vi "Pixie4ReadRunStatistics.vi"(8 "error in (no error)":errorcluster) -> (0 "error out":errorcluster, 2 "Run time [s]":dbl, 3 "run data output":T1, 5 "number of events":dbl)   [LabVIEW 2016]
uses:
  Drivers/Pixie4DLL.dll
panel:
  in  "run data":T1
  in  "Module number":u16 max=17 step=1
  in  "Run statistics":enum32{"Channel", "Module"}(tab)
  out "GDT3":dbl
  out "GDT2":dbl
  out "GDT1":dbl
  out "GDT0":dbl
  out "GateRate3":dbl
  out "GateRate2":dbl
  out "GateRate1":dbl
  out "GateRate0":dbl
  out "SFDT3":dbl
  out "SFDT2":dbl
  out "SFDT1":dbl
  out "SFDT0":dbl
  out "OCR3":dbl
  out "OCR2":dbl
  out "OCR1":dbl
  out "OCR0":dbl
  out "ICR3":dbl
  out "ICR2":dbl
  out "ICR1":dbl
  out "ICR0":dbl
  out "LT3":dbl
  out "LT2":dbl
  out "LT1":dbl
  out "LT0":dbl
  out "Total time [s]":dbl
  out "Event rate [cps]":dbl
  out "x/y":dbl
  # "Channel"
  # "Live time [s]"
  # "Input rates [cps]"
  # "Output rates [cps]"
  # "Filter dead time [s]"
  # "Gate rate [cps]"
  # "Gate dead time [s]"
  # "0"
  # "1"
  # "2"
  # "3"
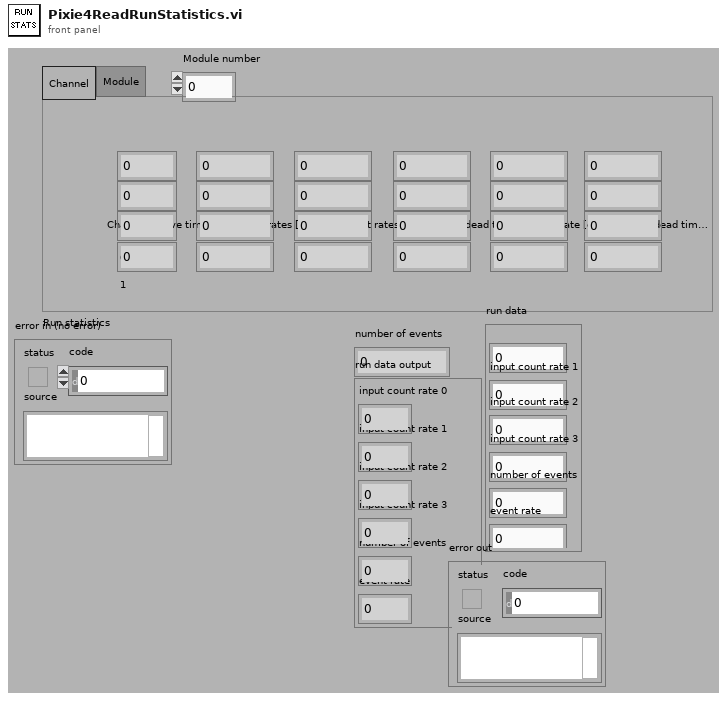
[diagram p1: front panel]
types:
  T1 = cluster{"input count rate 0":dbl, "input count rate 1":dbl, "input count rate 2":dbl, "input count rate 3":dbl, "number of events":dbl, "event rate":dbl}
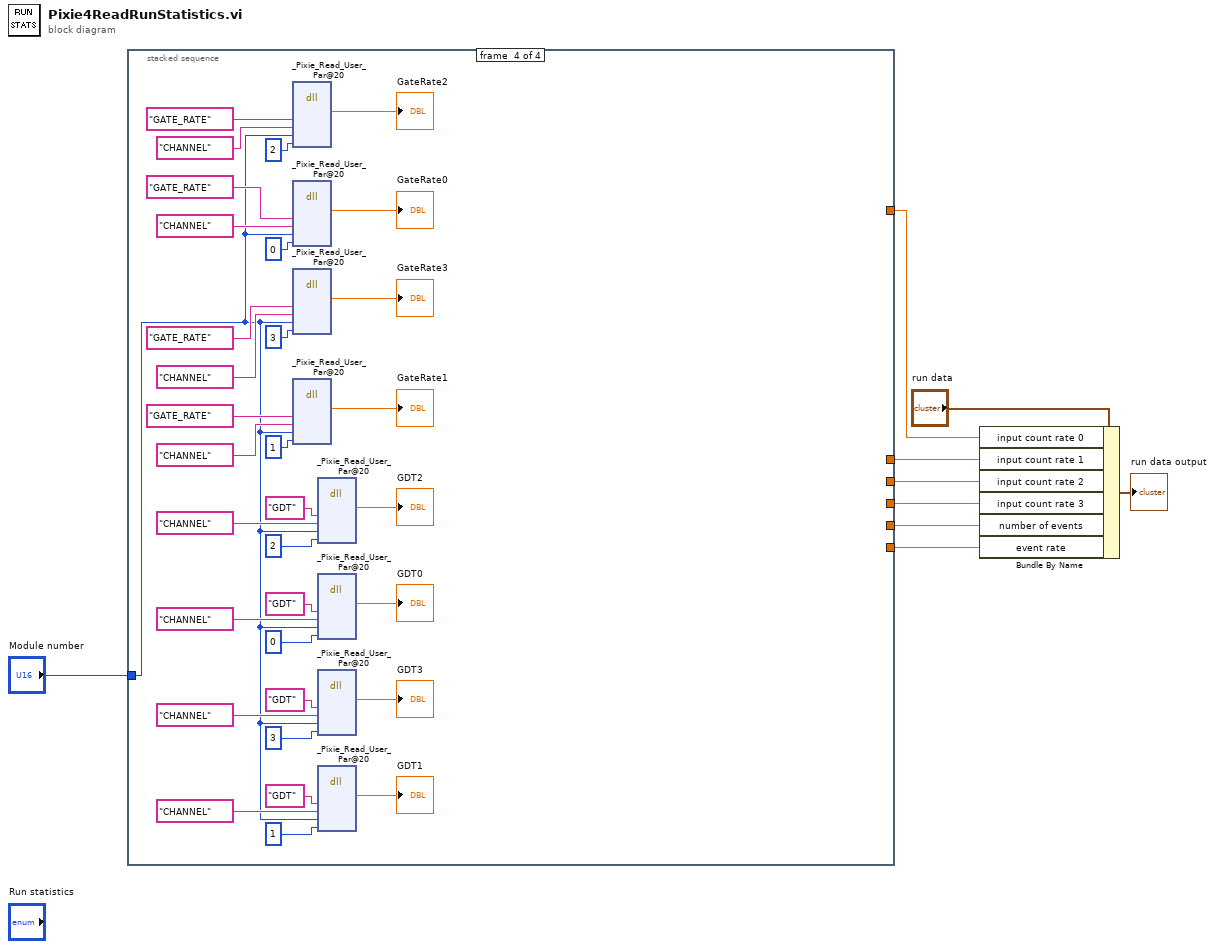
[diagram p0: block diagram]
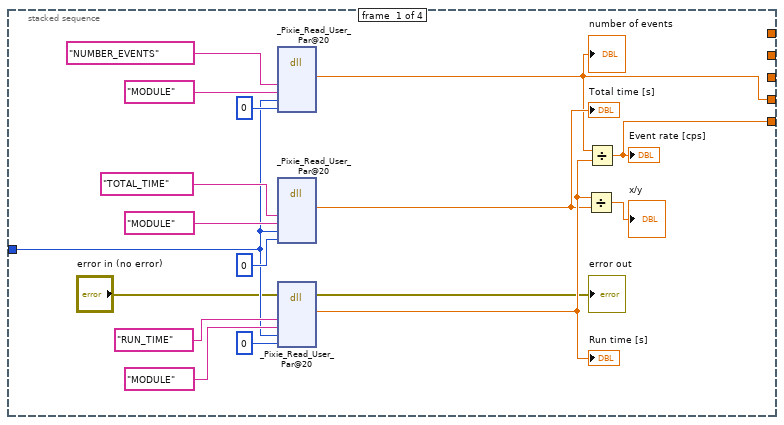
[diagram p2: hidden frame]
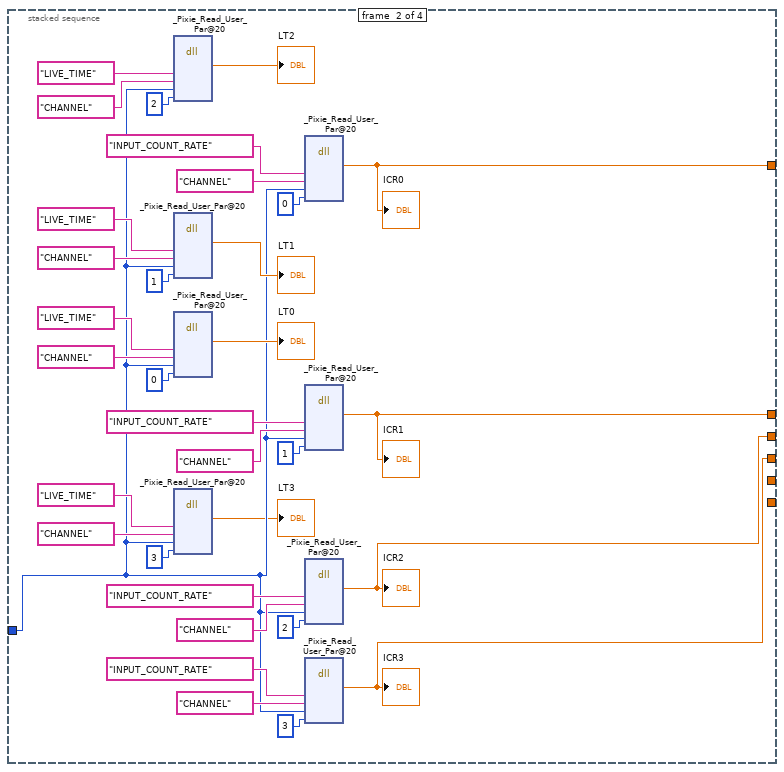
[diagram p3: hidden frame]
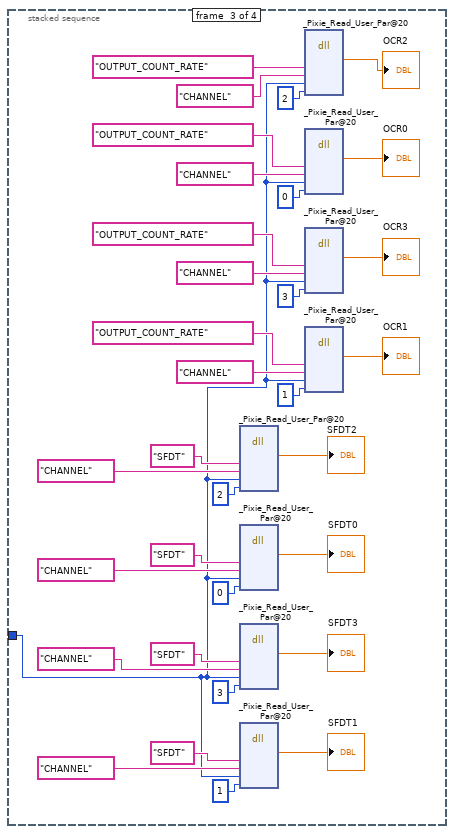
[diagram p4: hidden frame]
diagram:
  n1 = stacked-sequence {
    tunnel: "Module number" -> [w17 w32 w60 w93]
    tunnel: [_ w30 _ _] -> w7
    tunnel: [_ w29 _ _] -> w6
    tunnel: [_ w28 _ _] -> w5
    tunnel: [_ w27 _ _] -> w4
    tunnel: [w13 _ _ _] -> w3
    tunnel: [w12 _ _ _] -> w2
    frame #0 {
      n2 = dll-call lib="D:/Users/wymanm/Desktop/DAQuiri - 2017a/lois/Drivers/Pixie4DLL.dll" fn="_Pixie_Read_User_Par@20"("User_Par_Name"="NUMBER_EVENTS", "User_Par_Type"="MODULE", "ModNum"=w17, "ChanNum"=0) -> ("User_Par_Value"=w13:dbl)  [unwired: 9 in, 2 out]
      "number of events" <- w13
      n3 = dll-call lib="D:/Users/wymanm/Desktop/DAQuiri - 2017a/lois/Drivers/Pixie4DLL.dll" fn="_Pixie_Read_User_Par@20"("User_Par_Name"="TOTAL_TIME", "User_Par_Type"="MODULE", "ModNum"=w17, "ChanNum"=0) -> ("User_Par_Value"=w15:dbl)  [unwired: 9 in, 2 out]
      "Total time [s]" <- w15
      n4 = dll-call lib="D:/Users/wymanm/Desktop/DAQuiri - 2017a/lois/Drivers/Pixie4DLL.dll" fn="_Pixie_Read_User_Par@20"(error in="error in (no error)", "User_Par_Name"="RUN_TIME", "User_Par_Type"="MODULE", "ModNum"=w17, "ChanNum"=0) -> (error out=→"error out":errorcluster, "User_Par_Value"=w16:dbl)  [unwired: 8 in, 1 out]
      "Run time [s]" <- w16
      n5 = Divide(x=w16, y=w15) -> (x/y=→"x/y":dbl)
      n6 = Divide(x=w13, y=w16) -> (x/y=w12:dbl)
      "Event rate [cps]" <- w12
    }
    frame #1 {
      n7 = dll-call lib="D:/Users/wymanm/Desktop/DAQuiri - 2017a/lois/Drivers/Pixie4DLL.dll" fn="_Pixie_Read_User_Par@20"("User_Par_Name"="LIVE_TIME", "User_Par_Type"="CHANNEL", "ModNum"=w32, "ChanNum"=2) -> ("User_Par_Value"=→"LT2":dbl)  [unwired: 9 in, 2 out]
      n8 = dll-call lib="D:/Users/wymanm/Desktop/DAQuiri - 2017a/lois/Drivers/Pixie4DLL.dll" fn="_Pixie_Read_User_Par@20"("User_Par_Name"="LIVE_TIME", "User_Par_Type"="CHANNEL", "ModNum"=w32, "ChanNum"=1) -> ("User_Par_Value"=→"LT1":dbl)  [unwired: 9 in, 2 out]
      n9 = dll-call lib="D:/Users/wymanm/Desktop/DAQuiri - 2017a/lois/Drivers/Pixie4DLL.dll" fn="_Pixie_Read_User_Par@20"("User_Par_Name"="LIVE_TIME", "User_Par_Type"="CHANNEL", "ModNum"=w32, "ChanNum"=0) -> ("User_Par_Value"=→"LT0":dbl)  [unwired: 9 in, 2 out]
      n10 = dll-call lib="D:/Users/wymanm/Desktop/DAQuiri - 2017a/lois/Drivers/Pixie4DLL.dll" fn="_Pixie_Read_User_Par@20"("User_Par_Name"="LIVE_TIME", "User_Par_Type"="CHANNEL", "ModNum"=w32, "ChanNum"=3) -> ("User_Par_Value"=→"LT3":dbl)  [unwired: 9 in, 2 out]
      n11 = dll-call lib="D:/Users/wymanm/Desktop/DAQuiri - 2017a/lois/Drivers/Pixie4DLL.dll" fn="_Pixie_Read_User_Par@20"("User_Par_Name"="INPUT_COUNT_RATE", "User_Par_Type"="CHANNEL", "ModNum"=w32, "ChanNum"=0) -> ("User_Par_Value"=w30:dbl)  [unwired: 9 in, 2 out]
      "ICR0" <- w30
      n12 = dll-call lib="D:/Users/wymanm/Desktop/DAQuiri - 2017a/lois/Drivers/Pixie4DLL.dll" fn="_Pixie_Read_User_Par@20"("User_Par_Name"="INPUT_COUNT_RATE", "User_Par_Type"="CHANNEL", "ModNum"=w32, "ChanNum"=1) -> ("User_Par_Value"=w29:dbl)  [unwired: 9 in, 2 out]
      "ICR1" <- w29
      n13 = dll-call lib="D:/Users/wymanm/Desktop/DAQuiri - 2017a/lois/Drivers/Pixie4DLL.dll" fn="_Pixie_Read_User_Par@20"("User_Par_Name"="INPUT_COUNT_RATE", "User_Par_Type"="CHANNEL", "ModNum"=w32, "ChanNum"=2) -> ("User_Par_Value"=w28:dbl)  [unwired: 9 in, 2 out]
      "ICR2" <- w28
      n14 = dll-call lib="D:/Users/wymanm/Desktop/DAQuiri - 2017a/lois/Drivers/Pixie4DLL.dll" fn="_Pixie_Read_User_Par@20"("User_Par_Name"="INPUT_COUNT_RATE", "User_Par_Type"="CHANNEL", "ModNum"=w32, "ChanNum"=3) -> ("User_Par_Value"=w27:dbl)  [unwired: 9 in, 2 out]
      "ICR3" <- w27
    }
    frame #2 {
      n15 = dll-call lib="D:/Users/wymanm/Desktop/DAQuiri - 2017a/lois/Drivers/Pixie4DLL.dll" fn="_Pixie_Read_User_Par@20"("User_Par_Name"="SFDT", "User_Par_Type"="CHANNEL", "ModNum"=w60, "ChanNum"=2) -> ("User_Par_Value"=→"SFDT2":dbl)  [unwired: 9 in, 2 out]
      n16 = dll-call lib="D:/Users/wymanm/Desktop/DAQuiri - 2017a/lois/Drivers/Pixie4DLL.dll" fn="_Pixie_Read_User_Par@20"("User_Par_Name"="SFDT", "User_Par_Type"="CHANNEL", "ModNum"=w60, "ChanNum"=0) -> ("User_Par_Value"=→"SFDT0":dbl)  [unwired: 9 in, 2 out]
      n17 = dll-call lib="D:/Users/wymanm/Desktop/DAQuiri - 2017a/lois/Drivers/Pixie4DLL.dll" fn="_Pixie_Read_User_Par@20"("User_Par_Name"="SFDT", "User_Par_Type"="CHANNEL", "ModNum"=w60, "ChanNum"=3) -> ("User_Par_Value"=→"SFDT3":dbl)  [unwired: 9 in, 2 out]
      n18 = dll-call lib="D:/Users/wymanm/Desktop/DAQuiri - 2017a/lois/Drivers/Pixie4DLL.dll" fn="_Pixie_Read_User_Par@20"("User_Par_Name"="SFDT", "User_Par_Type"="CHANNEL", "ModNum"=w60, "ChanNum"=1) -> ("User_Par_Value"=→"SFDT1":dbl)  [unwired: 9 in, 2 out]
      n19 = dll-call lib="D:/Users/wymanm/Desktop/DAQuiri - 2017a/lois/Drivers/Pixie4DLL.dll" fn="_Pixie_Read_User_Par@20"("User_Par_Name"="OUTPUT_COUNT_RATE", "User_Par_Type"="CHANNEL", "ModNum"=w60, "ChanNum"=2) -> ("User_Par_Value"=→"OCR2":dbl)  [unwired: 9 in, 2 out]
      n20 = dll-call lib="D:/Users/wymanm/Desktop/DAQuiri - 2017a/lois/Drivers/Pixie4DLL.dll" fn="_Pixie_Read_User_Par@20"("User_Par_Name"="OUTPUT_COUNT_RATE", "User_Par_Type"="CHANNEL", "ModNum"=w60, "ChanNum"=0) -> ("User_Par_Value"=→"OCR0":dbl)  [unwired: 9 in, 2 out]
      n21 = dll-call lib="D:/Users/wymanm/Desktop/DAQuiri - 2017a/lois/Drivers/Pixie4DLL.dll" fn="_Pixie_Read_User_Par@20"("User_Par_Name"="OUTPUT_COUNT_RATE", "User_Par_Type"="CHANNEL", "ModNum"=w60, "ChanNum"=3) -> ("User_Par_Value"=→"OCR3":dbl)  [unwired: 9 in, 2 out]
      n22 = dll-call lib="D:/Users/wymanm/Desktop/DAQuiri - 2017a/lois/Drivers/Pixie4DLL.dll" fn="_Pixie_Read_User_Par@20"("User_Par_Name"="OUTPUT_COUNT_RATE", "User_Par_Type"="CHANNEL", "ModNum"=w60, "ChanNum"=1) -> ("User_Par_Value"=→"OCR1":dbl)  [unwired: 9 in, 2 out]
    }
    frame #3 {
      n23 = dll-call lib="D:/Users/wymanm/Desktop/DAQuiri - 2017a/lois/Drivers/Pixie4DLL.dll" fn="_Pixie_Read_User_Par@20"("User_Par_Name"="GATE_RATE", "User_Par_Type"="CHANNEL", "ModNum"=w93, "ChanNum"=2) -> ("User_Par_Value"=→"GateRate2":dbl)  [unwired: 9 in, 2 out]
      n24 = dll-call lib="D:/Users/wymanm/Desktop/DAQuiri - 2017a/lois/Drivers/Pixie4DLL.dll" fn="_Pixie_Read_User_Par@20"("User_Par_Name"="GATE_RATE", "User_Par_Type"="CHANNEL", "ModNum"=w93, "ChanNum"=0) -> ("User_Par_Value"=→"GateRate0":dbl)  [unwired: 9 in, 2 out]
      n25 = dll-call lib="D:/Users/wymanm/Desktop/DAQuiri - 2017a/lois/Drivers/Pixie4DLL.dll" fn="_Pixie_Read_User_Par@20"("User_Par_Name"="GATE_RATE", "User_Par_Type"="CHANNEL", "ModNum"=w93, "ChanNum"=3) -> ("User_Par_Value"=→"GateRate3":dbl)  [unwired: 9 in, 2 out]
      n26 = dll-call lib="D:/Users/wymanm/Desktop/DAQuiri - 2017a/lois/Drivers/Pixie4DLL.dll" fn="_Pixie_Read_User_Par@20"("User_Par_Name"="GATE_RATE", "User_Par_Type"="CHANNEL", "ModNum"=w93, "ChanNum"=1) -> ("User_Par_Value"=→"GateRate1":dbl)  [unwired: 9 in, 2 out]
      n27 = dll-call lib="D:/Users/wymanm/Desktop/DAQuiri - 2017a/lois/Drivers/Pixie4DLL.dll" fn="_Pixie_Read_User_Par@20"("User_Par_Name"="GDT", "User_Par_Type"="CHANNEL", "ModNum"=w93, "ChanNum"=2) -> ("User_Par_Value"=→"GDT2":dbl)  [unwired: 9 in, 2 out]
      n28 = dll-call lib="D:/Users/wymanm/Desktop/DAQuiri - 2017a/lois/Drivers/Pixie4DLL.dll" fn="_Pixie_Read_User_Par@20"("User_Par_Name"="GDT", "User_Par_Type"="CHANNEL", "ModNum"=w93, "ChanNum"=0) -> ("User_Par_Value"=→"GDT0":dbl)  [unwired: 9 in, 2 out]
      n29 = dll-call lib="D:/Users/wymanm/Desktop/DAQuiri - 2017a/lois/Drivers/Pixie4DLL.dll" fn="_Pixie_Read_User_Par@20"("User_Par_Name"="GDT", "User_Par_Type"="CHANNEL", "ModNum"=w93, "ChanNum"=3) -> ("User_Par_Value"=→"GDT3":dbl)  [unwired: 9 in, 2 out]
      n30 = dll-call lib="D:/Users/wymanm/Desktop/DAQuiri - 2017a/lois/Drivers/Pixie4DLL.dll" fn="_Pixie_Read_User_Par@20"("User_Par_Name"="GDT", "User_Par_Type"="CHANNEL", "ModNum"=w93, "ChanNum"=1) -> ("User_Par_Value"=→"GDT1":dbl)  [unwired: 9 in, 2 out]
    }
  }
  n31 = Bundle By Name(cluster="run data", "input count rate 0"=w7, "input count rate 1"=w6, "input count rate 2"=w5, "input count rate 3"=w4, "number of events"=w3, "event rate"=w2) -> (→"run data output":T1)
